vi "init.vi"(8 "error in (no error)":errorcluster, 11 "vehicleGeneric in":refnum<class "vehicleGeneric.lvclass">) -> (0 "error out":errorcluster, 3 "vehicleGeneric out":refnum<class "vehicleGeneric.lvclass">)   [LabVIEW 2011, in "vehicleGeneric.lvclass"]
uses:
  vehicleGeneric.lvclass
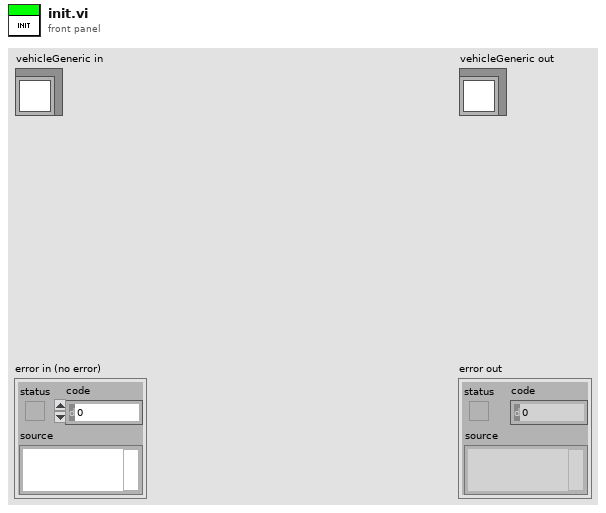
[diagram p1: front panel]
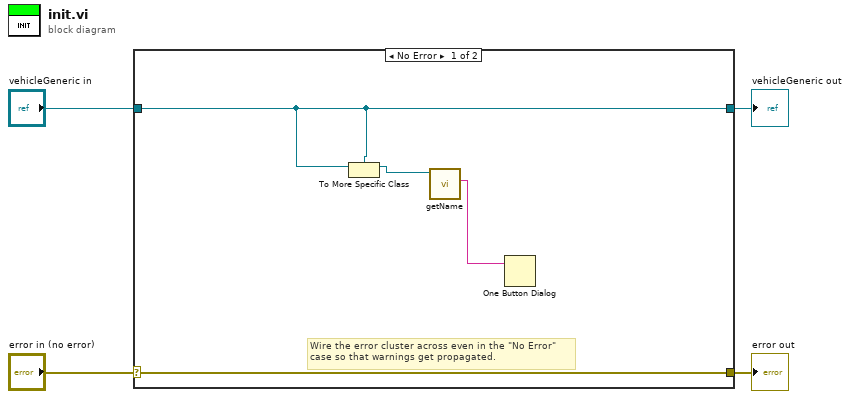
[diagram p0: block diagram]
diagram:
  n1 = case shown="No Error" "error in (no error)" {
    selector: "error in (no error)" -> [w8 w10]
    tunnel: [w8 w10] -> w3
    tunnel: [w7 w9] -> w1
    tunnel: "vehicleGeneric in" -> [w7 w9]
    frame No Error {
      # "Wire the error cluster across even in the \"No Error\"\ncase so that warnings get propagated."
      n2 = To More Specific Class(target class=w7, reference=w7) -> (specific class reference=w6:refnum<class "vehicleGeneric.lvclass">)  [unwired: 1 in, 1 out]
      n3 = call-dynamic "getName.vi"("vehicleGeneric in"=w6) -> ("name"=w5:string)  [unwired: 8 in, 2 out]
      n4 = One Button Dialog(message=w5) -> ()  [unwired: 1 in, 1 out]
    }
    frame Error {
    }
  }
  "error out" <- w3
  "vehicleGeneric out" <- w1
